vi "Test App Get Process After Stopping App.vi"(8 "error in (no error)":errorcluster, 11 "Rig Test in":refnum<class "Application Dev Test.lvclass">) -> (0 "error out":errorcluster, 3 "Rig Test out":refnum<class "Application Dev Test.lvclass">)   [LabVIEW 2020, in "Application Dev Test.lvclass"]
uses:
  Application Dev Test.lvclass
  C:/Program Files (x86)/National Instruments/LabVIEW 2020/vi.lib/Astemes/LUnit/Test Case.lvclass
  source/Framework/Process/Process.lvclass
  source/Framework/Process/Process.lvclass/Process.ctl
  source/Framework/Application/Application.lvclass/Application.ctl
  <vilib>/Astemes/LUnit/Test Case.lvclass/Test Case.ctl
  source/Framework/Application/Private/Add Process to Map.vi
  source/Framework/Application/Private/Throw Error If Process Already in App.vi
  source/Framework/Process/Protected/Messaging/Send Message.vi
  source/Framework/Process/Public/Lifecycle/Get Lifecycle State.vi
  source/Framework/Process/Protected/SubVIs/Set Context.vi
  source/Framework/Process/Private/SubVIs/Wait for finish.vi
  source/Framework/Process/Private/SubVIs/Set Lifecycle State.vi
  source/Framework/Application/Private/Retrieve Process from App.vi
  source/Framework/Application/Private/Parse Process Name.vi
  source/Framework/Application/Private/Get Process from Map.vi
  <vilib>/Astemes/LUnit/Palette/Fail.vi
  <vilib>/Astemes/LUnit/Palette/Pass.vi
  <vilib>/Astemes/LUnit/Set Assertion Type.vi
  source/Framework/Process/Private/SubVIs/Handle Debug Data.vi
  <vilib>/Utility/error.llb/Clear Errors.vi
  source/Framework/Process/Public/Lifecycle/Leave Process Loop.vi
  source/Framework/Process/Protected/Messaging/Request Message.vi
  <vilib>/AdvancedString/Delimited String to 1D String Array.vi
  <vilib>/Astemes/LUnit/Add test result.vi
  source/Framework/Logging/Log Debug.vi
  <vilib>/AdvancedString/1D String Array to Delimited String.vi
  <vilib>/Utility/High Resolution Relative Seconds.vi
  source/Framework/Process/Private/SubVIs/Enqueue Request Message.vi
  <vilib>/Astemes/LUnit/LUnit Record Assertion Result.vi
  <vilib>/Astemes/LUnit/LUnit Aggregate Assertion Results.vi
  <vilib>/Astemes/LUnit/Method Result/LUnit Merge Status.vi
  <vilib>/Astemes/LUnit/LUnit Concatenate result strings.vi
  source/Framework/Application/Application.lvclass
  C:/Git/astemes-triarc-framework/source/Framework/Process/Process.lvclass
  <vilib>/Utility/error.llb/Error Cluster From Error Code.vi
  source/Framework/Process/Private/SubVIs/Wait for Response Message.vi
  <vilib>/Astemes/LUnit/Test Case.lvclass
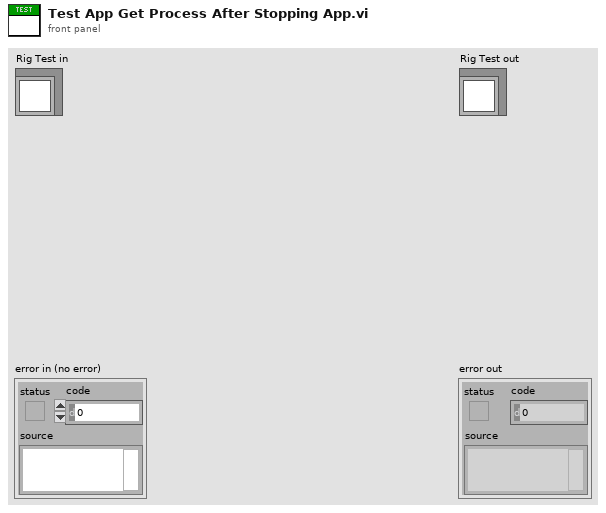
[diagram p1: front panel]
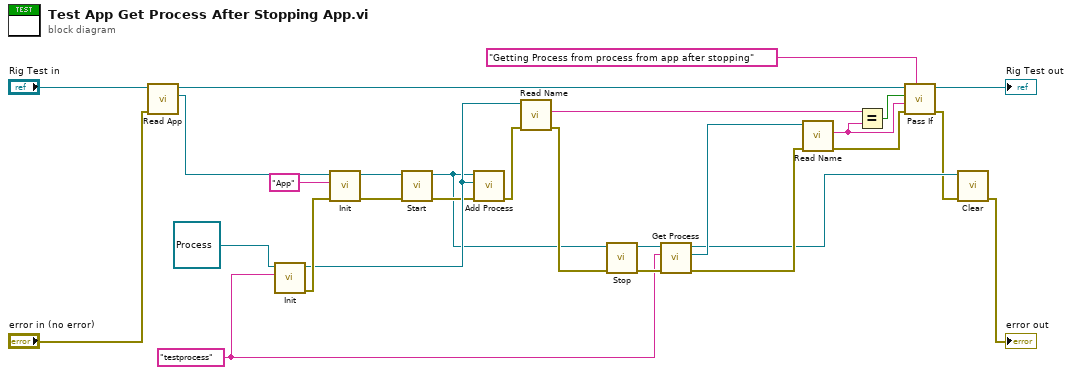
[diagram p0: block diagram]
diagram:
  w2 = "testprocess" ("Name")
  n1 = call "Read App.vi"("error in (no error)"="error in (no error)", "Application Test In"="Rig Test in") -> ("App out"=w27:refnum<class "Application.lvclass">, "Application Test Out"=w19:refnum<class "Application Dev Test.lvclass">)  [unwired: 7 in, 1 out]
  n2 = call-dynamic "Init.vi"("Name"=w2, "Process In"=refnum<class "Process.lvclass"> refnum ("Process.lvclass")) -> ("error out"=w18:errorcluster, "Process Out"=w8:refnum<class "Process.lvclass">)  [unwired: 8 in]
  n3 = call-dynamic "Init.vi"("error in (no error)"=w18, "Name"="App", "Process In"=w27) -> ("error out"=w21:errorcluster, "Process Out"=w5:refnum<class "Application.lvclass">)  [unwired: 7 in]
  n4 = call "Start.vi"("error in (no error)"=w21, "Process In"=w5) -> ("error out"=w6:errorcluster, "Process Out"=w1:refnum<class "Application.lvclass">)  [unwired: 7 in, 1 out]
  n5 = call "Add Process.vi"("error in (no error)"=w6, "Process"=w8, "Application In"=w1) -> ("error out"=w4:errorcluster)  [unwired: 7 in, 1 out]
  n6 = call "Read Name.vi"("error in (no error)"=w4, "Process In"=w8) -> ("error out"=w3:errorcluster, "Qualified Name"=w7:string)  [unwired: 6 in, 2 out]
  n7 = call "Stop.vi"("error in (no error)"=w3, "Process In"=w1) -> ("error out"=w22:errorcluster, "Process Out"=w23:refnum<class "Application.lvclass">)  [unwired: 7 in, 1 out]
  n8 = call "Get Process.vi"("error in (no error)"=w22, "Process Name"=w2, "Application In"=w23) -> ("error out"=w13:errorcluster, "App Process"=w16:refnum<class "Process.lvclass">, "Application Out"=w11:refnum<class "Application.lvclass">)  [unwired: 6 in]
  n9 = call "Read Name.vi"("error in (no error)"=w13, "Process In"=w16) -> ("error out"=w12:errorcluster, "Qualified Name"=w14:string)  [unwired: 6 in, 2 out]
  n10 = Equal?(x=w7, y=w14) -> (x = y?=w15:bool)
  n11 = call <vilib>:"Pass If.vi"("Description"="Getting Process from process from app after stopping", "error in (no error)"=w12, "Message"=w14, "Pass?"=w15, "LUnit Test Case In"=w19) -> ("error out"=w10:errorcluster, "LUnit Test Case Out"=→"Rig Test out":refnum<class "Application Dev Test.lvclass">)  [unwired: 5 in]
  n12 = call-dynamic "Clear.vi"("error in (no error)"=w10, "Application In"=w11) -> ("error out"=→"error out":errorcluster)  [unwired: 9 in]
